vi "Get_Client_Status_string.vi"(2 "Client State Cluster":T1={"Client Name"="", "Traverse level State"=enum."Complete", "People to Email"=[], "Next Contact Time"=0.0}, 3 "Client Name":string) -> (0 "Code Value":dbl=14.0 format="%.2f")   [LabVIEW 2010]
uses:
  ADAM Client/Sub VIs/ADAM Controls/Client_State_Cluster.ctl
  ADAM Client/Sub VIs/ADAM Controls/Traverse_Level_State.ctl
  ADAM Client/Sub VIs/ADAM Controls/Remember_value_mode.ctl
  ADAM_Global.vi
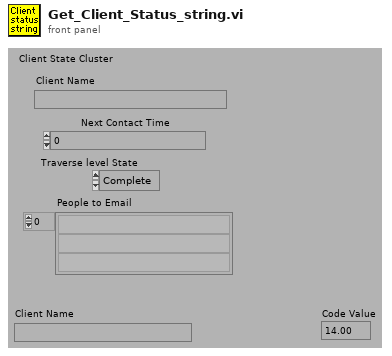
[diagram p1: front panel]
types:
  T1 = typedef "Client_State_Cluster.ctl" = cluster{"Client Name":string, "Traverse level State":T2, "People to Email":string[], "Next Contact Time":dbl}
  T2 = typedef "Traverse_Level_State.ctl" = enum16{"Running", "Complete"}
  T3 = typedef "Remember_value_mode.ctl" = enum16{"Read only", "Read and Write"}
  T4 = enum16{"Highest", "High", "Normal", "Low", "Lowest"}
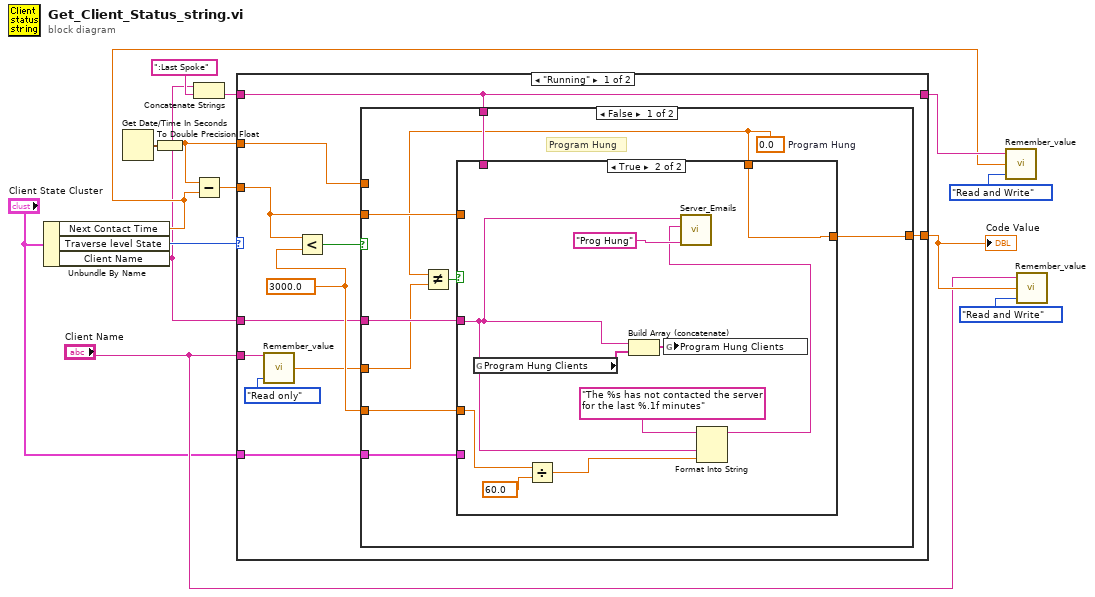
[diagram p0: block diagram]
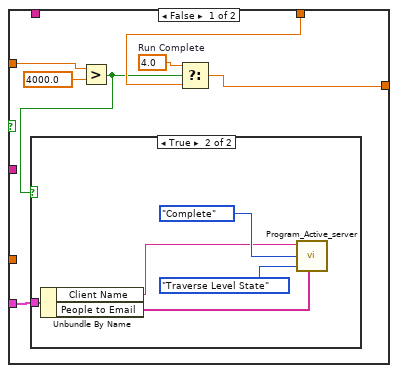
[diagram p2: hidden frame]
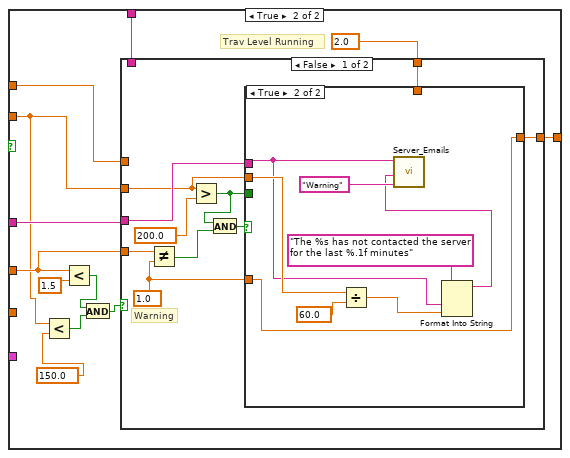
[diagram p4: hidden frame]
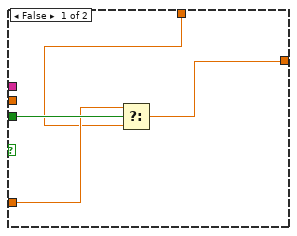
[diagram p5: hidden frame]
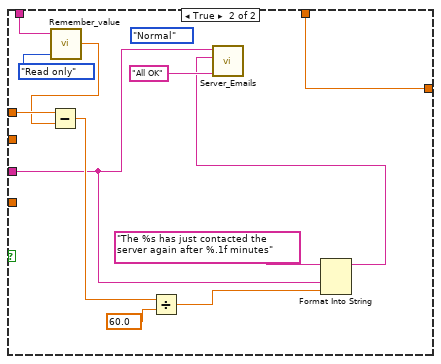
[diagram p6: hidden frame]
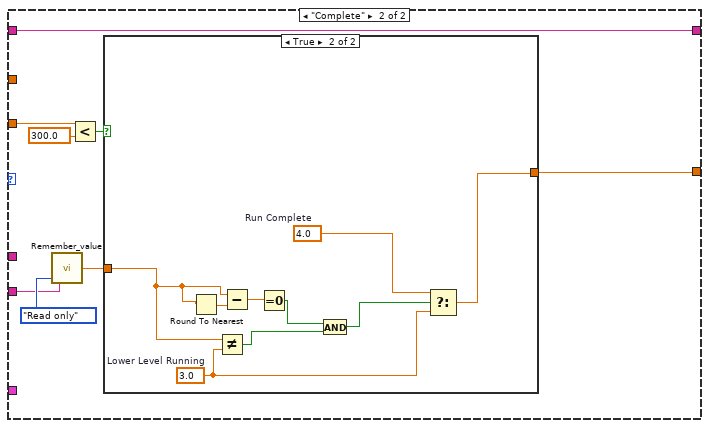
[diagram p7: hidden frame]
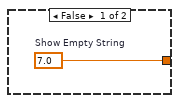
[diagram p8: hidden frame]
diagram:
  n1 = Unbundle By Name("Client State Cluster") -> ("Next Contact Time"=w5:dbl, "Traverse level State"=w3:T2, "Client Name"=w2:string)
  n2 = Get Date/Time In Seconds() -> (seconds since 1Jan1904=w1:timestamp)
  n3 = To Double Precision Float(number=w1) -> (double precision float=w12:dbl)
  n4 = Concatenate Strings(w2, ":Last Spoke" ("Substring")) -> (w7:string)
  n5 = Subtract(x=w12, y=w5) -> (x-y=w11:dbl)
  n6 = case shown="\"Running\"" w3 {
    tunnel: w12 -> [w17 _]
    tunnel: [w24 w104] -> w13
    tunnel: "Client Name" -> [w20 w106]
    tunnel: w11 -> [w16 w110]
    tunnel: w2 -> [w22 _]
    tunnel: [w18 w103] -> w6
    tunnel: w7 -> [w18 w103]
    tunnel: "Client State Cluster" -> [w15 _]
    frame "Running" {
      w23 = 3000.0 ("y")
      n7 = call "Remember_value.vi"("Mode"=Remember_value_mode."Read only", "Ch name"=w20) -> ("Output Value"=w19:dbl)  [unwired: 1 in]
      n8 = Less?(x=w16, y=w23) -> (x < y?=w25:bool)
      n9 = case shown="False" w25 {
        tunnel: [w28 w65] -> w24
        tunnel: w23 -> [w33 _]
        tunnel: w22 -> [w32 w68]
        tunnel: w19 -> [w31 w63]
        tunnel: w18 -> [w30 w67]
        tunnel: w17 -> [_ w66]
        tunnel: w16 -> [w29 w61]
        tunnel: w15 -> [w26 _]
        frame False {
          w27 = 0.0  # Program Hung
          # "Program Hung"
          n10 = Not Equal?(x=w27, y=w31) -> (x != y?=w34:bool)
          n11 = case shown="True" w34 {
            tunnel: w32 -> [_ w47]
            tunnel: w33 -> [_ w50]
            tunnel: w30 -> [_ _]
            tunnel: w29 -> [w41 _]
            tunnel: [w37 w53] -> w28
            tunnel: w27 -> [w39 w53]
            tunnel: w26 -> [w36 _]
            frame False {
              w38 = 4.0  # Run Complete
              n12 = Greater?(x=w41, y=4000.0) -> (0:w35:bool)
              n13 = case shown="True" w35 {
                tunnel: w36 -> [_ w46]
                frame False {
                }
                frame True {
                  n14 = Unbundle By Name(w46) -> ("Client Name"=w42:string, "People to Email"=w45:string[])
                  n15 = call "Program_Active_server.vi"("Client Name"=w42, "Traverse level State"=Traverse_Level_State."Complete", "Mode"=enum16{"Program Active", "Traverse Level State"}."Traverse Level State", "People to Email"=w45) -> ()  [unwired: 2 in, 5 out]
                }
              }
              n16 = Select(t=w38, s=w35, f=w39) -> (s? t:f=w37:dbl)
            }
            frame True {
              n17 = global read "ADAM_Global.vi" "Program Hung Clients"() -> (w49:string[])
              n18 = Divide(x=w50, y=60.0) -> (x/y=w52:dbl)
              n19 = Build Array (concatenate)(w47, w49) -> (w48:string[])
              n20 = global write "ADAM_Global.vi" "Program Hung Clients"(w48) -> ()
              n21 = Format Into String(format string="The %s has not contacted the server for the last %.1f minutes" ("Format String"), w47, w52) -> (resulting string=w54:string)  [unwired: 2 in, 1 out]
              n22 = call "Server_Emails.vi"("Client Name Contains"=w47, "Message"=w54, "Subject"="Prog Hung") -> ()  [unwired: 2 in, 3 out]
            }
          }
        }
        frame True {
          # "Trav Level Running"
          n23 = Less?(x=w61, y=150.0) -> (x < y?=w58:bool)
          n24 = Less?(x=w63, y=1.5) -> (x < y?=w59:bool)
          n25 = And(x=w59, y=w58) -> (x .and. y?=w57:bool)
          n26 = case shown="False" w57 {
            tunnel: w68 -> [w72 w91]
            tunnel: w67 -> [_ w100]
            tunnel: w66 -> [_ w99]
            tunnel: w61 -> [w69 _]
            tunnel: 2.0 ("y") -> [w78 w97]
            tunnel: [w77 w97] -> w65
            tunnel: w63 -> [w75 _]
            frame False {
              w71 = 1.0 ("y")
              # "Warning"
              n27 = Not Equal?(x=w75, y=w71) -> (x != y?=w74:bool)
              n28 = Greater?(x=w69, y=200.0) -> (0:w70:bool)
              n29 = And(x=w70, y=w74) -> (x .and. y?=w73:bool)
              n30 = case shown="True" w73 {
                tunnel: w78 -> [w80 _]
                tunnel: [w79 w89] -> w77
                tunnel: w69 -> [_ w85]
                tunnel: w72 -> [_ w83]
                tunnel: w70 -> [w82 _]
                tunnel: w71 -> [w81 w89]
                frame False {
                  n31 = Select(t=w81, s=w82, f=w80) -> (s? t:f=w79:dbl)
                }
                frame True {
                  n32 = Divide(x=w85, y=60.0) -> (x/y=w87:dbl)
                  n33 = Format Into String(format string="The %s has not contacted the server for the last %.1f minutes" ("Format String"), w83, w87) -> (resulting string=w84:string)  [unwired: 2 in, 1 out]
                  n34 = call "Server_Emails.vi"("Client Name Contains"=w83, "Message"=w84, "Subject"="Warning") -> ()  [unwired: 2 in, 3 out]
                }
              }
            }
            frame True {
              (unwired) T4."Normal" ("Priorities")
              n35 = call "Remember_value.vi"("Mode"=Remember_value_mode."Read only", "Ch name"=w100) -> ("Output Value"=w98:dbl)  [unwired: 1 in]
              n36 = Subtract(x=w99, y=w98) -> (x-y=w93:dbl)
              n37 = Divide(x=w93, y=60.0) -> (x/y=w95:dbl)
              n38 = Format Into String(format string="The %s has just contacted the server again after %.1f minutes" ("Format String"), w91, w95) -> (resulting string=w92:string)  [unwired: 2 in, 1 out]
              n39 = call "Server_Emails.vi"("Client Name Contains"=w91, "Message"=w92, "Subject"="All OK") -> ()  [unwired: 2 in, 3 out]
            }
          }
        }
      }
    }
    frame "Complete" {
      n40 = call "Remember_value.vi"("Mode"=Remember_value_mode."Read only", "Ch name"=w106) -> ("Output Value"=w105:dbl)  [unwired: 1 in]
      n41 = Less?(x=w110, y=300.0) -> (x < y?=w108:bool)
      n42 = case shown="True" w108 {
        tunnel: w105 -> [_ w116]
        tunnel: [w111 w117] -> w104
        frame False {
          w111 = 7.0  # Show Empty String
        }
        frame True {
          w118 = 4.0  # Run Complete
          w115 = 3.0  # Lower Level Running
          n43 = Round To Nearest(number=w116) -> (nearest integer value=w120:dbl)
          n44 = Not Equal?(x=w116, y=w115) -> (x != y?=w114:bool)
          n45 = Subtract(x=w116, y=w120) -> (x-y=w119:dbl)
          n46 = Equal To 0?(x=w119) -> (x = 0?=w113:bool)
          n47 = And(x=w113, y=w114) -> (x .and. y?=w112:bool)
          n48 = Select(t=w118, s=w112, f=w115) -> (s? t:f=w117:dbl)
        }
      }
    }
  }
  "Code Value" <- w13
  n49 = call "Remember_value.vi"("Mode"=Remember_value_mode."Read and Write", "Input Value"=w5, "Ch name"=w6) -> ()  [unwired: 1 out]
  n50 = call "Remember_value.vi"("Mode"=Remember_value_mode."Read and Write", "Input Value"=w13, "Ch name"="Client Name") -> ()  [unwired: 1 out]
